vi "WAPIErrorToAscii.vi"(8 "error in (no error)":errorcluster, 11 "error":u32) -> (0 "error out":errorcluster, 3 "psErr":string)   [LabVIEW 2009]
uses:
  win50032.dll
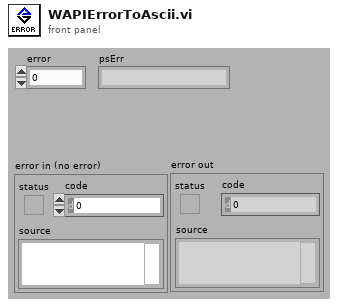
[diagram p1: front panel]
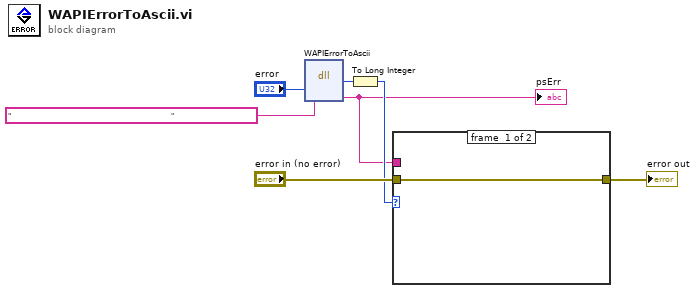
[diagram p0: block diagram]
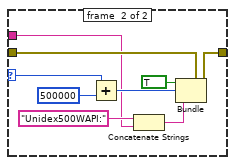
[diagram p2: hidden frame]
diagram:
  n1 = dll-call lib="win50032.dll" fn="WAPIErrorToAscii"("error"="error", "psErr"="                                                                                " ("error_string")) -> ("return type"=w4:u32, "psErr"=w2:string)  [unwired: 4 in, 2 out]
  "psErr" <- w2
  n2 = To Long Integer(number=w4) -> (32bit integer=w3:i32)
  n3 = case shown="0" w3 {
    selector: w3 -> [_ w10]
    tunnel: "error in (no error)" -> [w8 w17]
    tunnel: [w8 w16] -> w5
    tunnel: w2 -> [_ w9]
    frame #0 {
    }
    frame #1 {
      n4 = Add(x=w10, y=500000) -> (x+y=w12:i32)
      n5 = Concatenate Strings("Unidex500WAPI:" ("string"), w9) -> (w13:string)
      n6 = Bundle(cluster=w17, "status"=TRUE, "code"=w12, "source"=w13) -> (w16:errorcluster)
    }
  }
  "error out" <- w5
